vi "8byetcarray.vi"() -> ()   [LabVIEW 2014]
uses:
  <vilib>/Utility/file.llb/Write To Spreadsheet File (I64).vi
panel:
  out "Numeric":dbl
  out "Boolean":bool
  out "Slide":u32(slide) scale=0.0..250000.0
  in  "Path":path
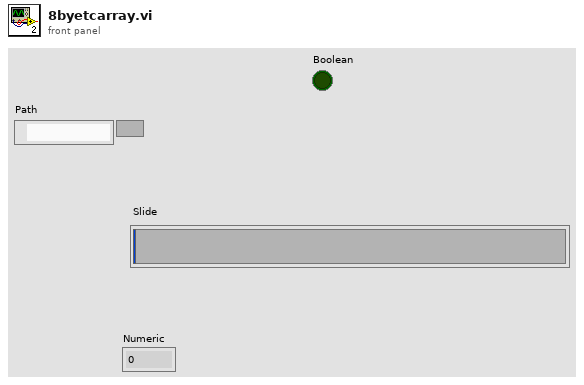
[diagram p1: front panel]
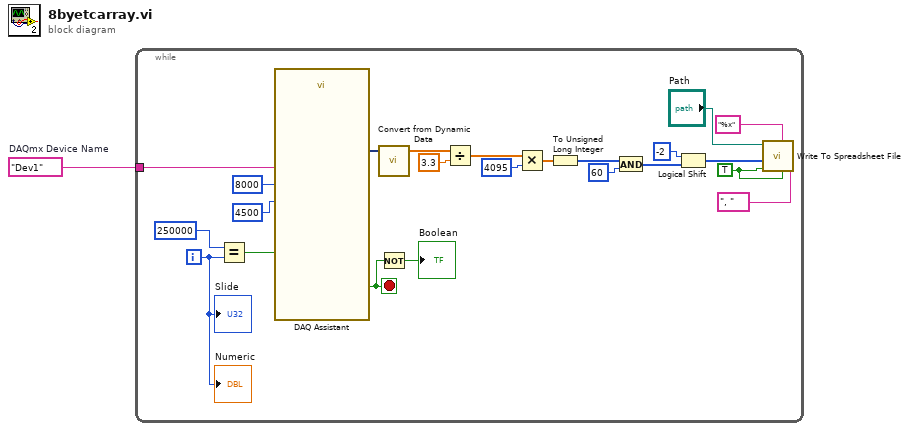
[diagram p0: block diagram]
diagram:
  w1 = tag "Dev1"  # DAQmx Device Name
  n1 = while {
    tunnel: w1 -> [w24]
    i -> [w2]
    stop <- w5 stop-if-true
    w3 = TRUE
    n2 = Equal?(x=250000, y=w2) -> (x = y?=w12:bool)
    n3 = call "DAQ Assistant"("rate"=4500, "number of samples"=8000, "stop (F)"=w12, "device name"=w24) -> ("data"=w14:dynamicdata, "stopped"=w5:bool)  [unwired: 12 in, 2 out]
    n4 = call "Convert from Dynamic Data"("Dynamic Data Type"=w14) -> ("Array"=w15:dbl[])  [unwired: 3 in]
    n5 = Not(x=w5) -> (.not. x?=→"Boolean":bool)
    n6 = Divide(x=w15, y=3.3) -> (x/y=w22:dbl[])
    n7 = Multiply(x=w22, y=4095) -> (x*y=w20:dbl[])
    n8 = To Unsigned Long Integer(number=w20) -> (unsigned 32bit integer=w19:u32[])
    n9 = And(x=w19, y=u32 60) -> (x .and. y?=w17:u32[])
    n10 = Logical Shift(y=-2, x=w17) -> (x << y=w8:u32[])
    n11 = call-poly <vilib>:"Write To Spreadsheet File.vi"("delimiter (\\t)"=", ", "transpose? (no:F)"=w3, "format (%d)"="%x", "append to file? (new file:F)"=w3, "1D data"=w8, "file path (dialog if empty)"="Path") -> ()  [unwired: 2 in, 1 out]
    "Slide" <- w2
    "Numeric" <- w2
  }
